vi "Cursors Page.vi"() -> ()   [LabVIEW 2020, in "2D Plot.lvclass"]
uses:
  <vilib>/Math Plots/2D Math Plots/2D Plot/2D Plot/2D Plot.lvclass
  <vilib>/Math Plots/2D Math Plots/2D Plot/Action String/2DMathPlot Ctrl Act Queue.ctl
  <vilib>/Math Plots/2D Math Plots/2D Plot/Action String/2DMathPlot Ctrl Act Cluster.ctl
  <vilib>/Math Plots/2D Math Plots/2D Plot/Action String/2DMathPlot State Class.ctl
  <vilib>/Math Plots/2D Math Plots/2D Plot/2D Plot/Typedef/Cursor Property.ctl
  <vilib>/Utility/miscctls.llb/LVCursorListTypeDef.ctl
  <vilib>/Math Plots/2D Math Plots/2D Plot/2D Plot/Typedef/Dialog State.ctl
  <vilib>/Math Plots/2D Math Plots/2D Plot/2D Plot/Typedef/Temp Graph State.ctl
panel:
  in  "Cursor":string="Cursors"
  in  "Plot # Prefix":string="All Plots"
  out "Cursor Property Out":T1
  in  "Cursor Property In":T1
  in  "Control Ref Queue":T3
  in  "Event Registration":refnum<event-registration>
  in  "Show Cursor":bool caption="Show name"
  in  "Line Width":T4 caption="Cursor Line Width"
  in  "Point Style":T5 caption="Cursor Point Style"
  in  "Line Style":T6 caption="Cursor Line Style"
  in  "Plot #":i32(ring) caption="Plot.Point Style" items=["All Plots", "Plot 0", ""]
  in  "Locking":i32(ring) caption="Plot.Line Width" items=["Free dragging", "Single-plot", "Multi-plot"]
  in  "Delete":bool
  in  "Add":bool
  in  "Show Name":bool caption="Show name"
  in  "Allow Dragging":bool caption="Allow dragging"
  in  "Cursor Name":string caption="Name"
  in  "Cursor Style":T7
  in  "Cursor Color":u32(colorbox) caption="Cursor color"
  in  "Active Cursor":i32(ring) caption="xActive Cursor"
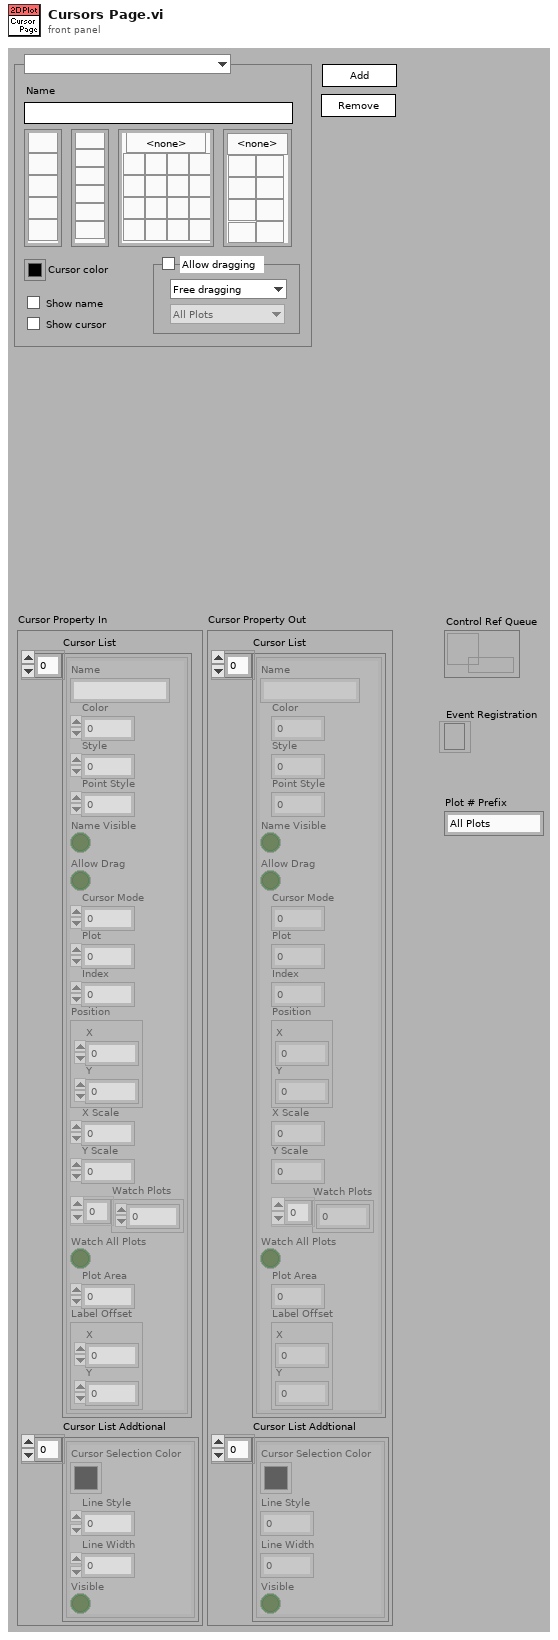
[diagram p1: front panel]
types:
  T1 = typedef "2D Plot.lvclass/Cursor Property.ctl" = cluster{"Cursor List":T2, "Cursor List Addtional":cluster{"Cursor Selection Color":u32, "Line Style":u8, "Line Width":u8, "Visible":bool}[]}
  T2 = typedef "LVCursorListTypeDef.ctl" = cluster{"Name":string, "Color":u32, "Style":u8, "Point Style":u8, "Name Visible":bool, "Allow Drag":bool, "Cursor Mode":u32, "Plot":i32, "Index":i32, "Position":cluster{"X":dbl, "Y":dbl}, "X Scale":u32, "Y Scale":u32, "Watch Plots":i32[], "Watch All Plots":bool, "Plot Area":i32, "Label Offset":cluster{"X":dbl, "Y":dbl}}[]
  T3 = typedef "2DMathPlot Ctrl Act Queue.ctl" = refnum<queue>
  T4 = cluster{"OK Button 2":bool, "OK Button 3":bool, "OK Button 4":bool, "OK Button 5":bool, "OK Button 6":bool, "OK Button 7":bool}
  T5 = cluster{"OK Button 17":bool, "OK Button":bool, "OK Button 2":bool, "OK Button 3":bool, "OK Button 4":bool, "OK Button 5":bool, "OK Button 6":bool, "OK Button 7":bool, "OK Button 8":bool, "OK Button 9":bool, "OK Button 10":bool, "OK Button 11":bool, "OK Button 12":bool, "OK Button 13":bool, "OK Button 14":bool, "OK Button 15":bool, "OK Button 16":bool}
  T6 = cluster{"OK Button":bool, "OK Button 2":bool, "OK Button 3":bool, "OK Button 4":bool, "OK Button 5":bool}
  T7 = cluster{"OK Button 17":bool, "OK Button":bool, "OK Button 2":bool, "OK Button 5":bool, "OK Button 13":bool, "OK Button 10":bool, "OK Button 6":bool, "OK Button 9":bool, "OK Button 14":bool}
  T8 = typedef "2D Plot.lvclass/Dialog State.ctl" = enum16{"Initialize", "Read Property", "Write Property", "Idle", "Exit"}
  T9 = typedef "2DMathPlot Ctrl Act Cluster.ctl" = cluster{"Plot Area Ref":refnum<vi>, "Z Axis Ref":refnum<vi>, "Legend Ref":refnum<vi>, "XControl Ref":refnum<vi>, "Facade Ref":refnum<vi>, "Display State Change Class":T10}
  T10 = typedef "2DMathPlot State Class.ctl" = enum16{"Update All (Undo)", "Update General", "Update Appearance", "Update Format", "Update Scale", "Update Marker", "Update Cursor", "None"}
  T11 = typedef "2D Plot.lvclass/Temp Graph State.ctl" = enum16{"Create", "Update Graph", "Update Property Only", "Get Plot Name", "Get Axis Name", "Destory"}
  T12 = cluster{"Cursor Selection Color":u32, "Line Style":u8, "Line Width":u8, "Visible":bool}
  T13 = cluster{"Name":string, "Color":u32, "Style":u8, "Point Style":u8, "Name Visible":bool, "Allow Drag":bool, "Cursor Mode":u32, "Plot":i32, "Index":i32, "Position":cluster{"X":dbl, "Y":dbl}, "X Scale":u32, "Y Scale":u32, "Watch Plots":i32[], "Watch All Plots":bool, "Plot Area":i32, "Label Offset":cluster{"X":dbl, "Y":dbl}}
  T14 = cluster{"Cursor Selection Color":u32, "Line Style":u8, "Line Width":u8, "Visible":bool}[]
  T15 = cluster{"Bool Array[0]":bool, "Bool Array[1]":bool, "Bool Array[2]":bool, "Bool Array[3]":bool, "Bool Array[4]":bool, "Bool Array[5]":bool, "Bool Array[6]":bool, "Bool Array[7]":bool, "Bool Array[8]":bool, "Bool Array[9]":bool, "Bool Array[10]":bool, "Bool Array[11]":bool, "Bool Array[12]":bool, "Bool Array[13]":bool, "Bool Array[14]":bool, "Bool Array[15]":bool, "Bool Array[16]":bool}
  T16 = cluster{"Bool Array[0]":bool, "Bool Array[1]":bool, "Bool Array[2]":bool, "Bool Array[3]":bool, "Bool Array[4]":bool, "Bool Array[5]":bool, "Bool Array[6]":bool, "Bool Array[7]":bool, "Bool Array[8]":bool}
  T17 = cluster{"Bool Array[0]":bool, "Bool Array[1]":bool, "Bool Array[2]":bool, "Bool Array[3]":bool, "Bool Array[4]":bool}
  T18 = cluster{"Bool Array[0]":bool, "Bool Array[1]":bool, "Bool Array[2]":bool, "Bool Array[3]":bool, "Bool Array[4]":bool, "Bool Array[5]":bool}
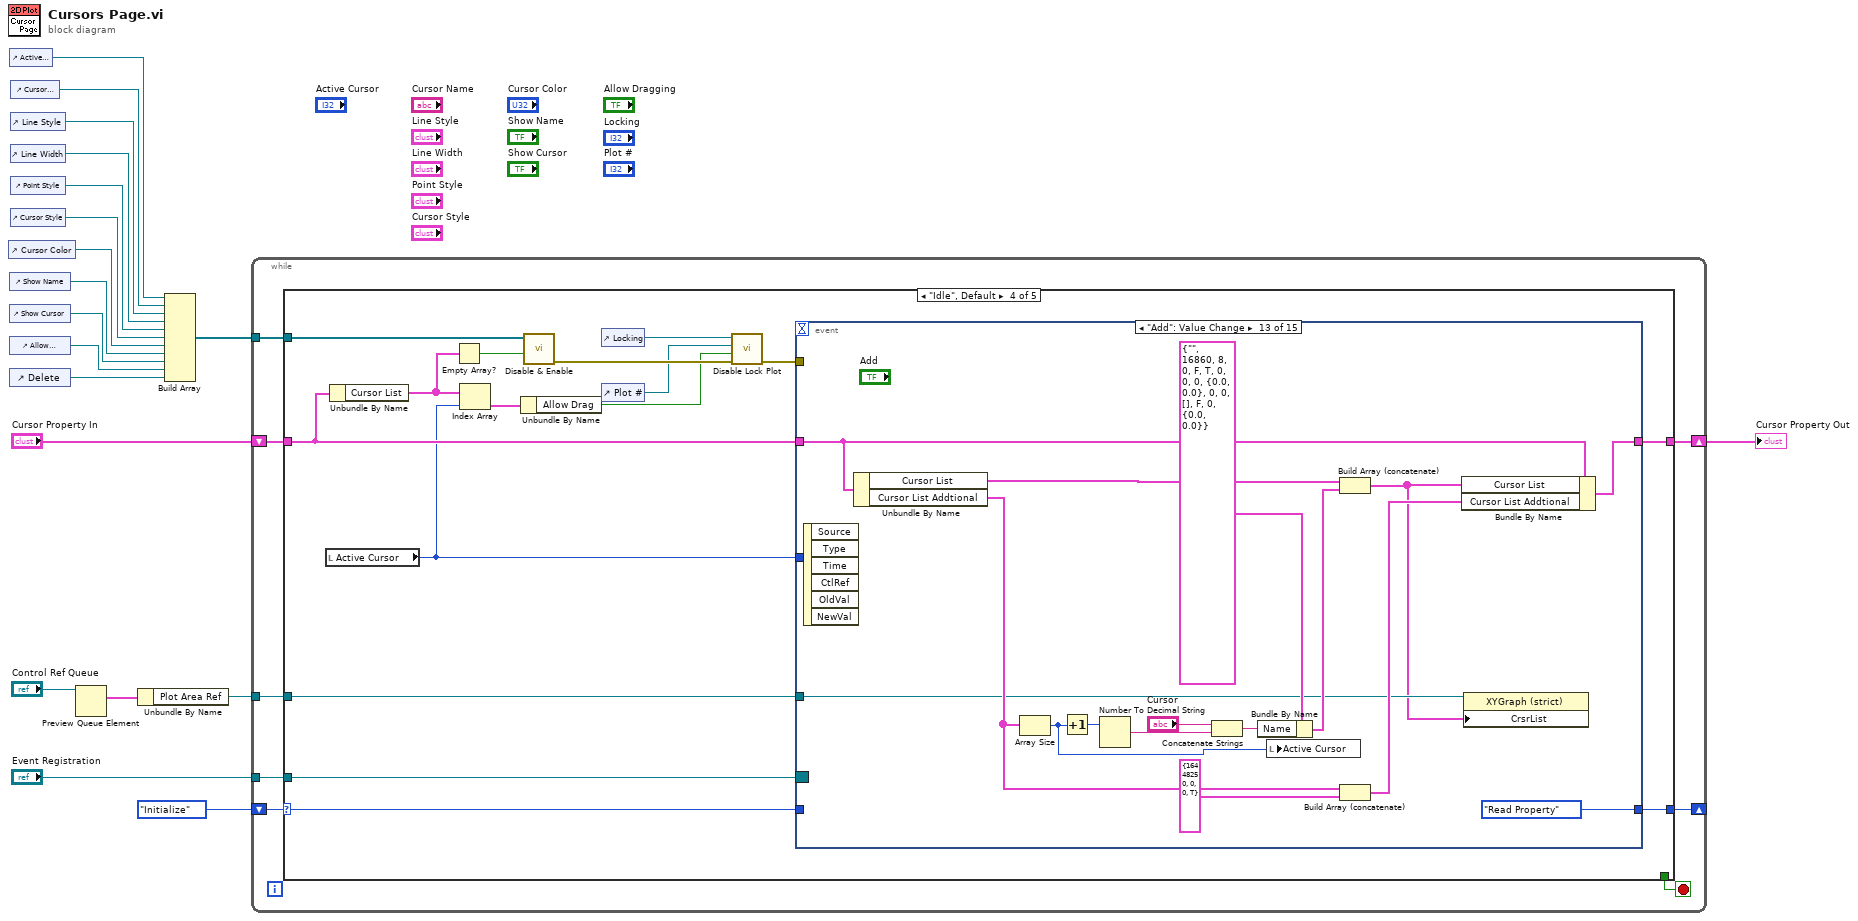
[diagram p0: block diagram]
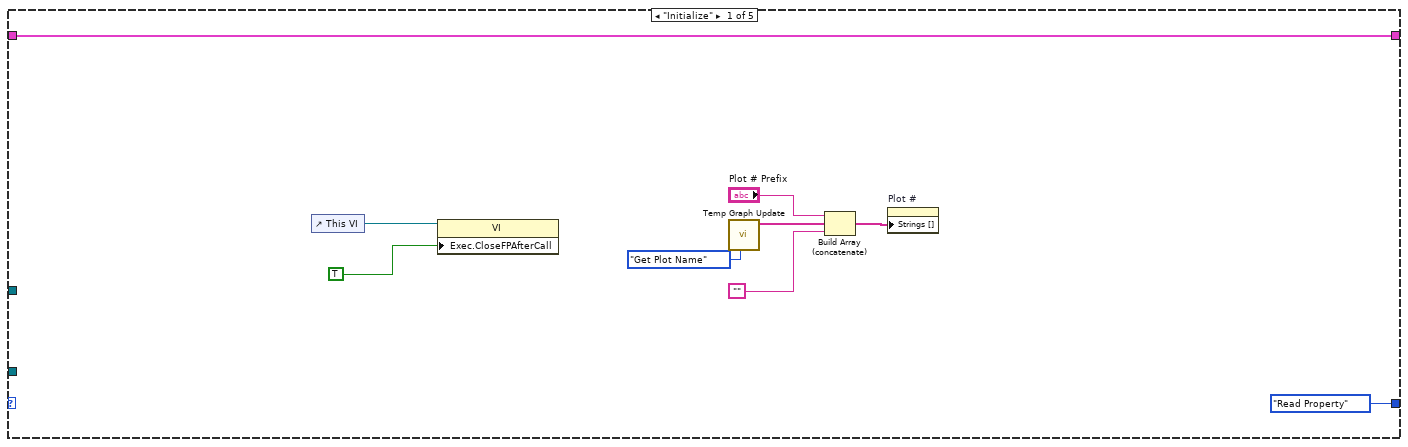
[diagram p2: hidden frame]
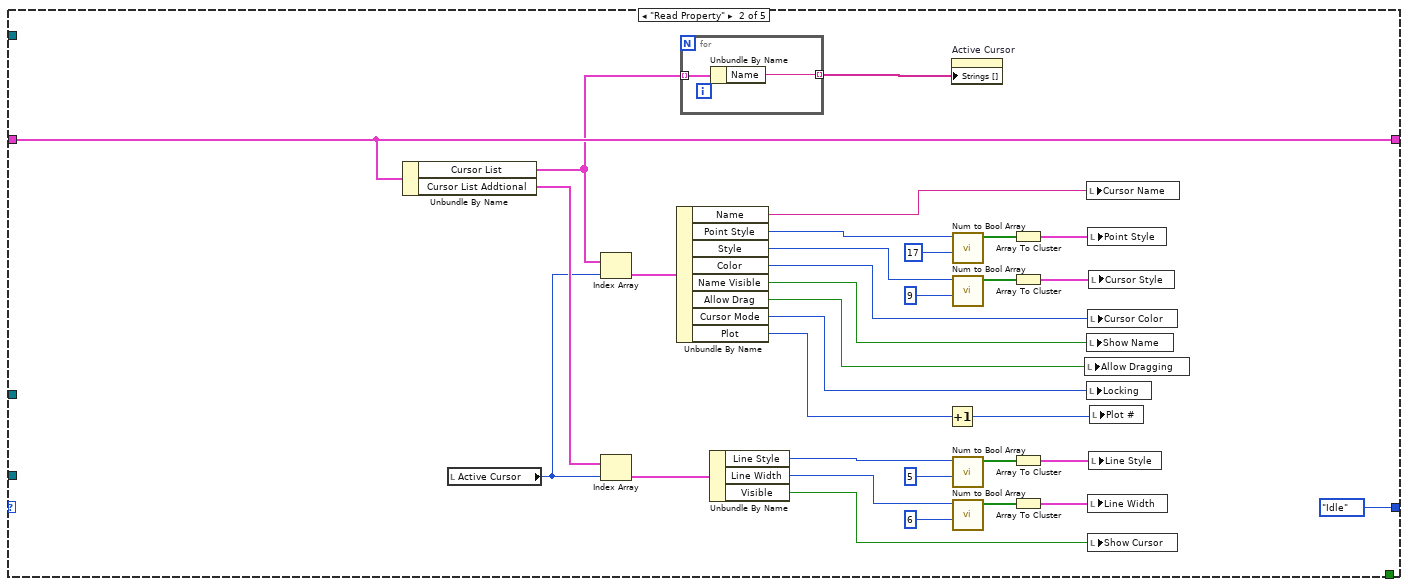
[diagram p3: hidden frame]
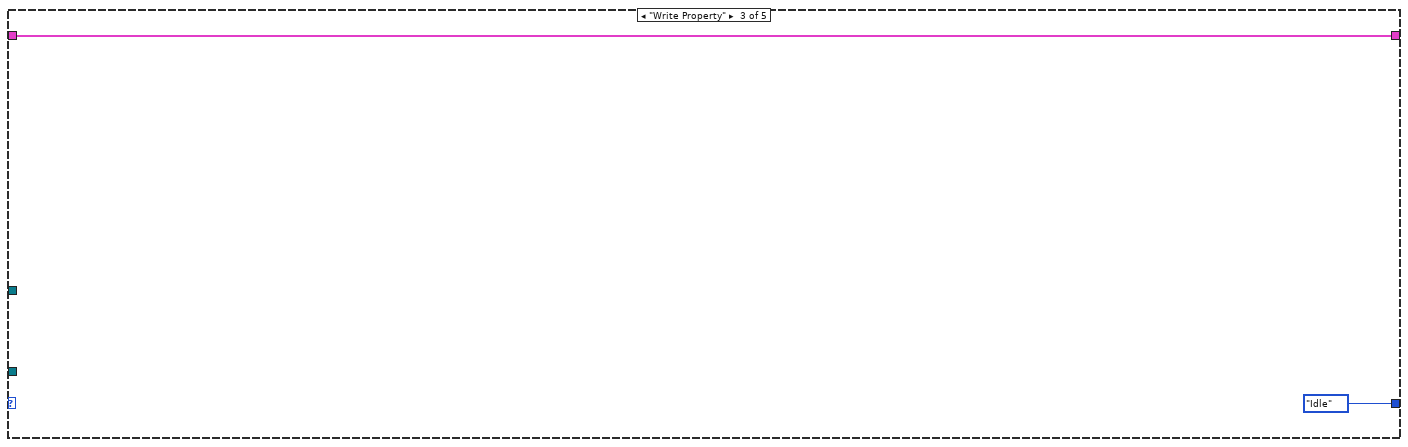
[diagram p4: hidden frame]
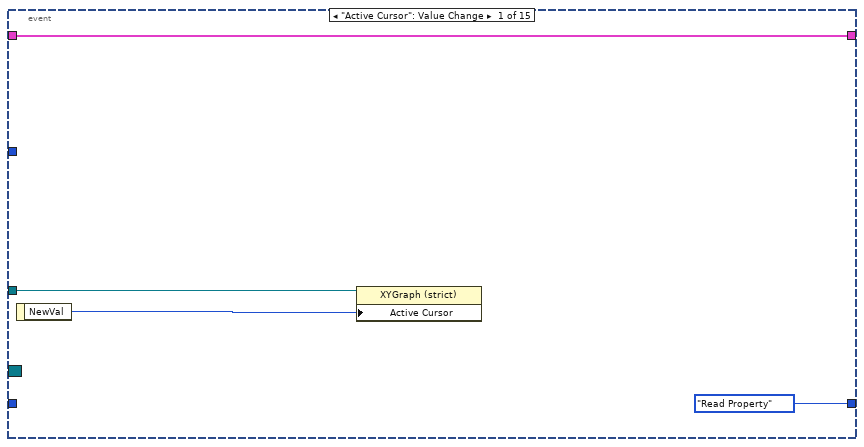
[diagram p5: hidden frame]
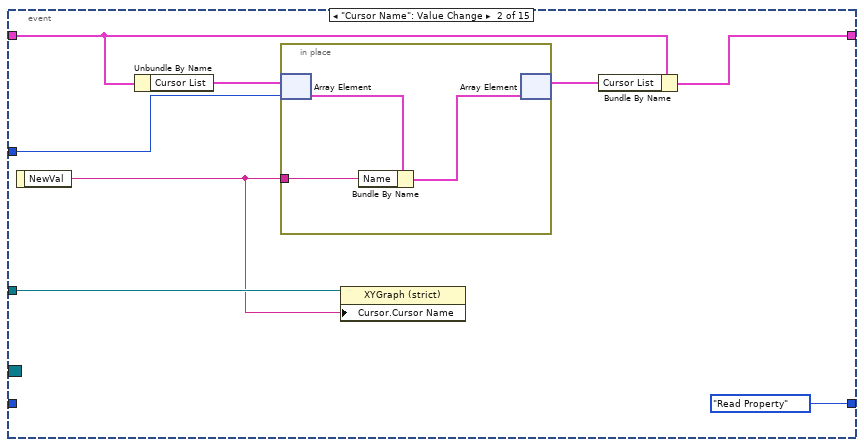
[diagram p6: hidden frame]
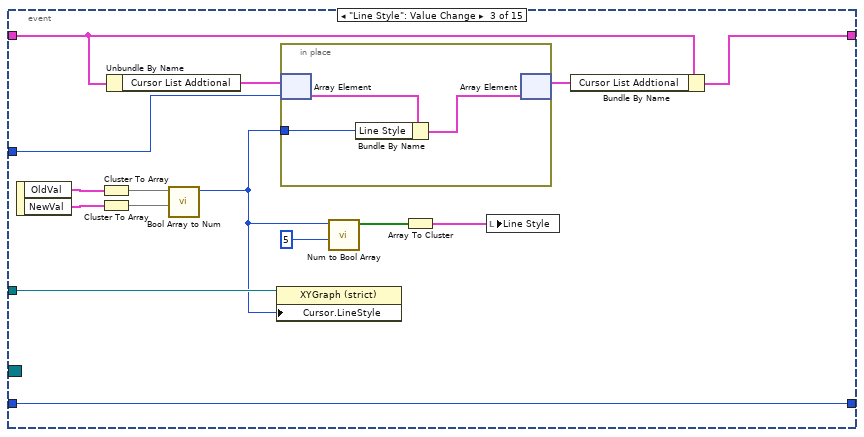
[diagram p7: hidden frame]
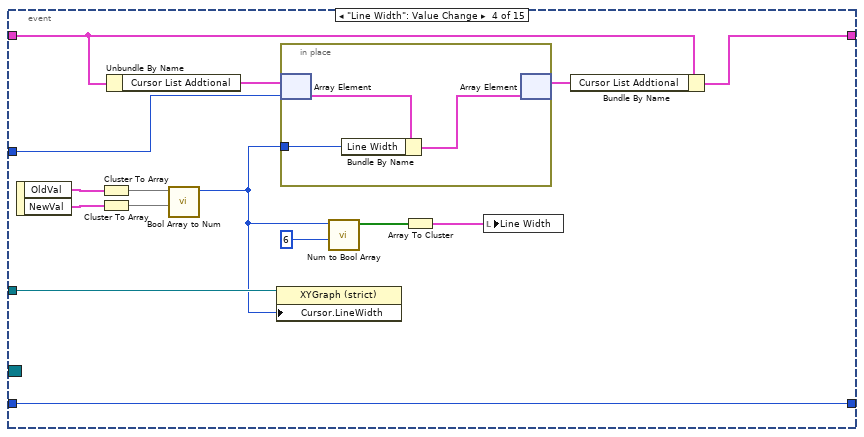
[diagram p8: hidden frame]
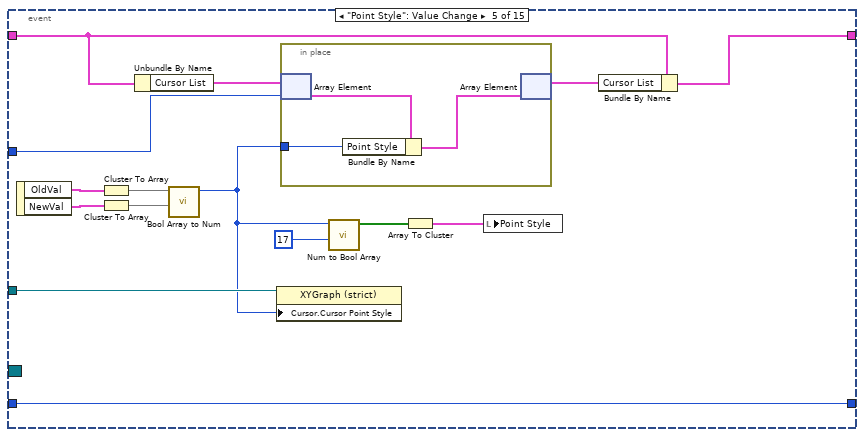
[diagram p9: hidden frame]
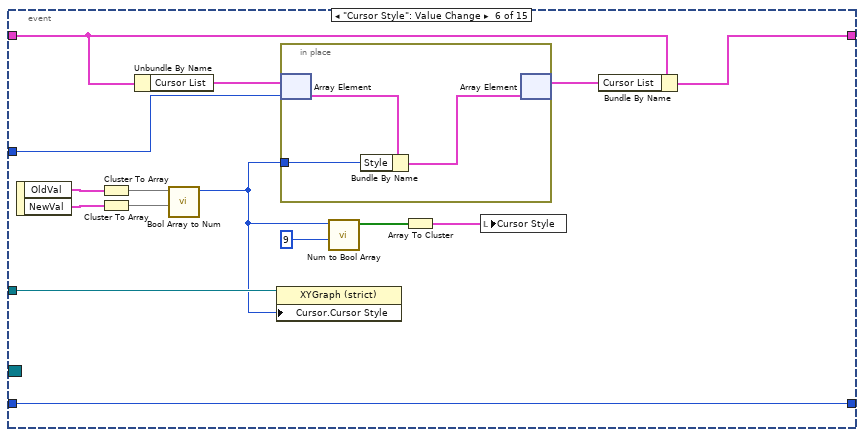
[diagram p10: hidden frame]
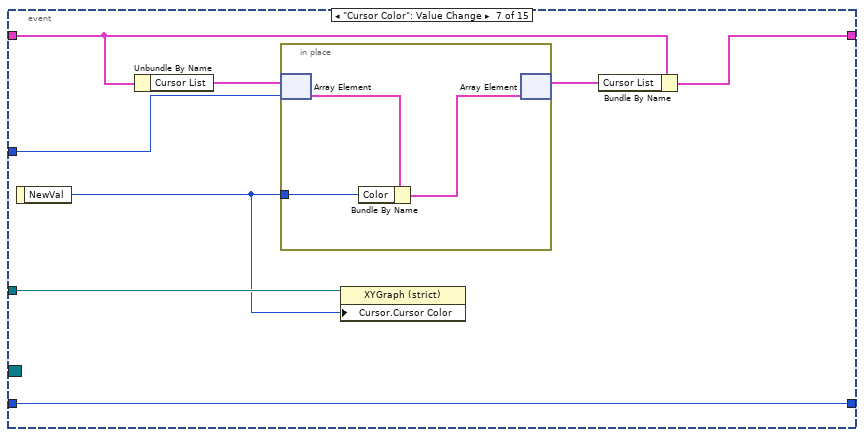
[diagram p11: hidden frame]
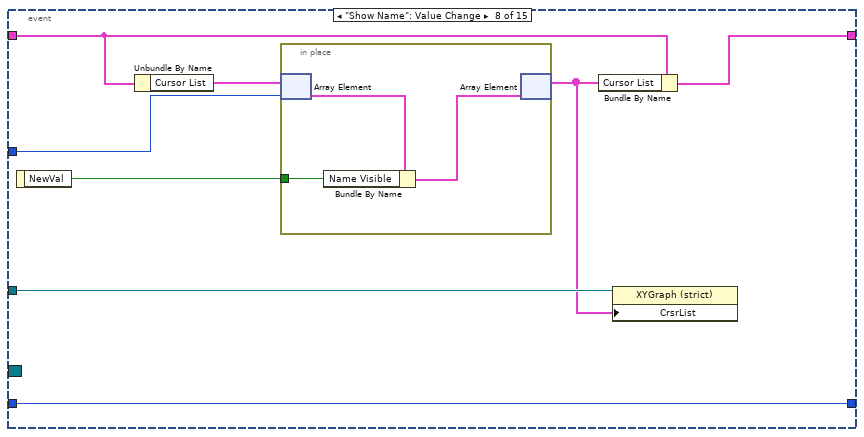
[diagram p12: hidden frame]
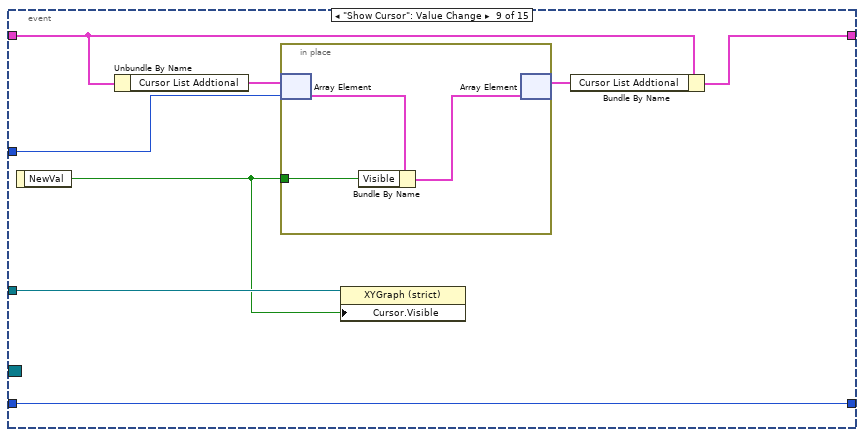
[diagram p13: hidden frame]
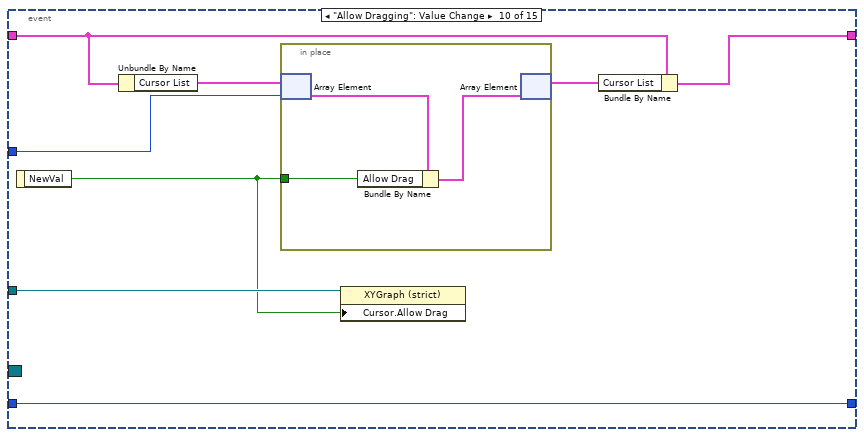
[diagram p14: hidden frame]
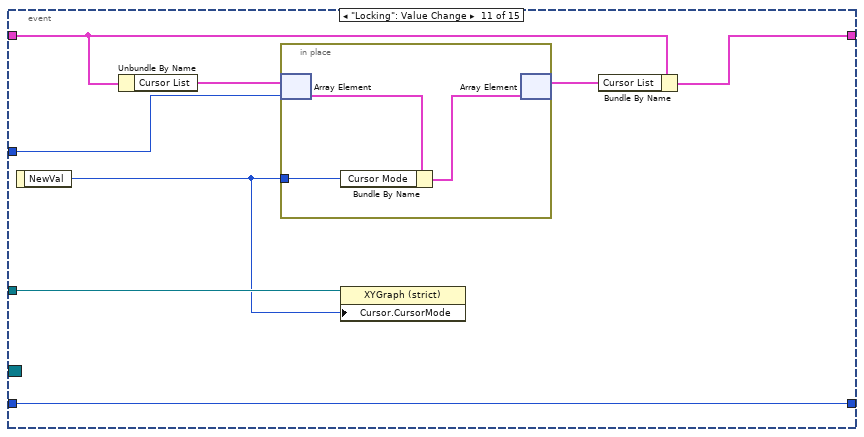
[diagram p15: hidden frame]
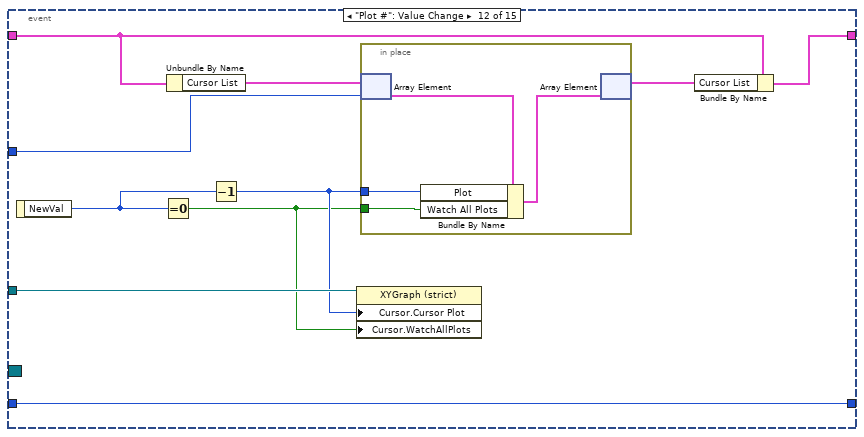
[diagram p16: hidden frame]
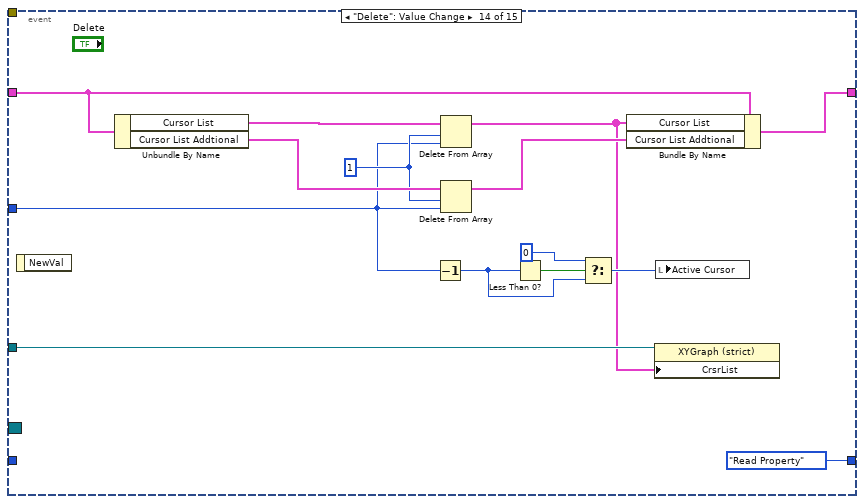
[diagram p17: hidden frame]
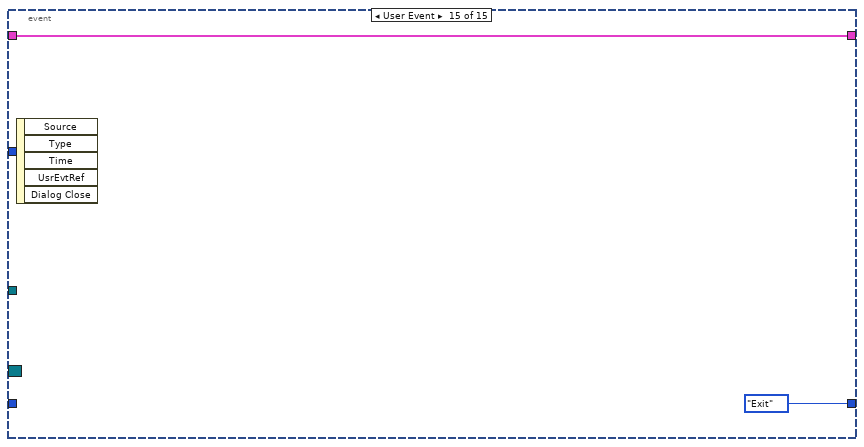
[diagram p18: hidden frame]
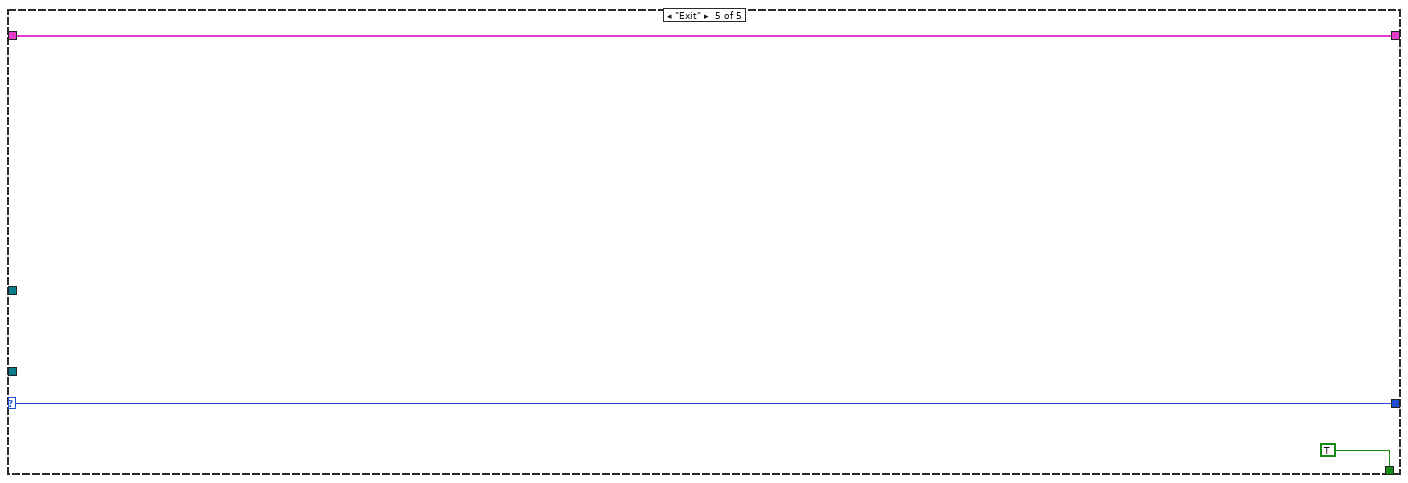
[diagram p19: hidden frame]
diagram:
  n1 = control-ref of="Cursor Color"() -> (w6:refnum<vi>)
  n2 = control-ref of="Active Cursor"() -> (w12:refnum<vi>)
  n3 = control-ref of="Show Name"() -> (w5:refnum<vi>)
  n4 = control-ref of="Show Cursor"() -> (w4:refnum<vi>)
  n5 = control-ref of="Allow Dragging"() -> (w3:refnum<vi>)
  n6 = control-ref of="Delete"() -> (w1:refnum<vi>)
  n7 = control-ref of="Cursor Name"() -> (w11:refnum<vi>)
  n8 = control-ref of="Line Style"() -> (w10:refnum<vi>)
  n9 = control-ref of="Line Width"() -> (w9:refnum<vi>)
  n10 = control-ref of="Point Style"() -> (w8:refnum<vi>)
  n11 = control-ref of="Cursor Style"() -> (w7:refnum<vi>)
  n12 = Preview Queue Element(queue="Control Ref Queue") -> (element=w19:T9)  [unwired: 1 in, 4 out]
  n13 = Unbundle By Name(w19) -> ("Plot Area Ref"=w16:refnum<vi>)
  n14 = Build Array(w12, w11, w10, w9, w8, w7, w6, w5, w4, w3, w1) -> (w2:refnum<vi>[])
  n15 = while {
    shift-right: [w24] -> _
    shift-left: Dialog_State."Initialize" ("Enum") -> [w27]
    tunnel: w16 -> [w26]
    tunnel: "Event Registration" -> [w25]
    shift-right: [w22] -> w13
    shift-left: "Cursor Property In" -> [w23]
    tunnel: w2 -> [w20]
    stop <- w21 stop-if-true
    n16 = case shown="\"Idle\", Default" w27 {
      selector: w27 -> [_ _ _ w84 w278]
      tunnel: w26 -> [_ _ _ w85 _]
      tunnel: w25 -> [_ _ _ w88 _]
      tunnel: [Dialog_State."Read Property" ("Enum") Dialog_State."Idle" ("Enum") Dialog_State."Idle" ("Enum") w87 w278] -> w24
      tunnel: w23 -> [w33 w62 w72 w82 w279]
      tunnel: [w33 w62 w72 w86 w279] -> w22
      tunnel: [_ _ _ _ TRUE] -> w21
      tunnel: w20 -> [_ _ _ w83 _]
      frame "Initialize" {
        n17 = control-ref of="This VI"() -> (w36:refnum<vi>)
        n18 = property class="VI"(reference=w36, "Exec.CloseFPAfterCall"=TRUE ("Execution:Close After Call")) -> ()  [unwired: 1 in, 2 out]
        n19 = call <vilib>:"Temp Graph Update.vi"("State"=Temp_Graph_State."Get Plot Name") -> ("Item Strings"=w29:string[])  [unwired: 4 in, 6 out]
        n20 = Build Array (concatenate)("Plot # Prefix", w29, "") -> (w30:string[])
        n21 = property on="Plot #" class="Ring (strict)"("Strings []"=w30) -> ()  [unwired: 2 in, 2 out]
      }
      frame "Read Property" {
        n22 = Unbundle By Name(w62) -> ("Cursor List"=w61:T2, "Cursor List Addtional"=w60:T14)
        n23 = local read "Active Cursor"() -> (w59:i32)
        n24 = Index Array(array=w61, index=w59) -> (element=w68:T13)
        n25 = Index Array(array=w60, index=w59) -> (element=w58:T12)
        n26 = Unbundle By Name(w68) -> ("Name"=w66:string, "Point Style"=w49:u8, "Style"=w45:u8, "Color"=w44:u32, "Name Visible"=w43:bool, "Allow Drag"=w42:bool, "Cursor Mode"=w41:u32, "Plot"=w39:i32)
        n27 = for {
          tunnel: w61 -> [w70] mode=indexing
          tunnel: [w69] -> w67 mode=indexing
          n28 = Unbundle By Name(w70) -> ("Name"=w69:string)
        }
        n29 = Unbundle By Name(w58) -> ("Line Style"=w57:u8, "Line Width"=w53:u8, "Visible"=w37:bool)
        n30 = Increment(x=w39) -> (x+1=w38:i32)
        n31 = property on="Active Cursor" class="Ring (strict)"("Strings []"=w67) -> ()  [unwired: 2 in, 2 out]
        n32 = call <vilib>:"Num to Bool Array.vi"("Array Size"=17, "Value"=w49) -> ("Bool Array"=w50:bool[])  [unwired: 9 out]
        n33 = call <vilib>:"Num to Bool Array.vi"("Array Size"=9, "Value"=w45) -> ("Bool Array"=w48:bool[])  [unwired: 9 out]
        n34 = call <vilib>:"Num to Bool Array.vi"("Array Size"=5, "Value"=w57) -> ("Bool Array"=w65:bool[])  [unwired: 9 out]
        n35 = call <vilib>:"Num to Bool Array.vi"("Array Size"=6, "Value"=w53) -> ("Bool Array"=w55:bool[])  [unwired: 9 out]
        n36 = Array To Cluster(array=w50) -> (cluster=w51:T15)
        n37 = Array To Cluster(array=w48) -> (cluster=w47:T16)
        n38 = Array To Cluster(array=w65) -> (cluster=w64:T17)
        n39 = Array To Cluster(array=w55) -> (cluster=w54:T18)
        n40 = local write "Allow Dragging"(w42) -> ()
        n41 = local write "Cursor Name"(w66) -> ()
        n42 = local write "Show Name"(w43) -> ()
        n43 = local write "Locking"(w41) -> ()
        n44 = local write "Point Style"(w51) -> ()
        n45 = local write "Cursor Color"(w44) -> ()
        n46 = local write "Line Width"(w54) -> ()
        n47 = local write "Show Cursor"(w37) -> ()
        n48 = local write "Cursor Style"(w47) -> ()
        n49 = local write "Line Style"(w64) -> ()
        n50 = local write "Plot #"(w38) -> ()
      }
      frame "Write Property" {
      }
      frame "Idle", Default {
        n51 = local read "Active Cursor"() -> (w78:i32)
        n52 = Unbundle By Name(w82) -> ("Cursor List"=w80:T2)
        n53 = Empty Array?(array=w80) -> (empty?=w81:bool)
        n54 = Index Array(array=w80, index=w78) -> (element=w79:T13)
        n55 = Unbundle By Name(w79) -> ("Allow Drag"=w76:bool)
        n56 = call <vilib>:"Disable & Enable.vi"("Disabled?"=w81, "Control Ref Array"=w83) -> ("error out"=w77:errorcluster)  [unwired: 1 in, 8 out]
        n57 = control-ref of="Locking"() -> (w75:refnum<vi>)
        n58 = control-ref of="Plot #"() -> (w74:refnum<vi>)
        n59 = call <vilib>:"Disable Lock Plot.vi"("error in (no error)"=w77, "Allow Drag"=w76, "Plot # Refnum"=w74, "Locking Refnum"=w75) -> ("error out"=w73:errorcluster)  [unwired: 7 out]
        n60 = event shown="[12] \"Add\": Value Change" {
          selector: w88 -> [_ _ _ _ _ _ _ _ _ _ _ _ _ _ _]
          dyn-events: _ -> [_ _ _ _ _ _ _ _ _ _ _ _ _ _ _]
          timeout: _ -> [_ _ _ _ _ _ _ _ _ _ _ _ _ _ _]
          tunnel: w82 -> [w91 w99 w117 w135 w153 w171 w182 w193 w204 w215 w226 w239 w259 w274 w276]
          tunnel: [Dialog_State."Read Property" ("Enum") Dialog_State."Read Property" ("Enum") w105 w123 w141 w159 w177 w191 w199 w210 w221 w235 Dialog_State."Read Property" ("Enum") Dialog_State."Read Property" ("Enum") Dialog_State."Exit" ("Enum")] -> w87
          tunnel: [w91 w97 w115 w133 w151 w169 w180 w192 w202 w213 w224 w237 w257 w273 w276] -> w86
          tunnel: w85 -> [w90 w96 w114 w132 w150 w168 w179 w188 w201 w212 w223 w236 w248 w262 _]
          tunnel: w84 -> [_ _ w105 w123 w141 w159 w177 w191 w199 w210 w221 w235 _ _ _]
          tunnel: w78 -> [_ w94 w104 w122 w140 w158 w176 w190 w198 w209 w220 w234 _ w264 _]
          tunnel: w73 -> [_ _ _ _ _ _ _ _ _ _ _ _ _ _ _]
          event "Active Cursor": Value Change {
            n61 = event-data() -> ("NewVal"=w89:i32)  [unwired: 1 out]
            n62 = property class="XYGraph (strict)"(reference=w90, "Active Cursor"=w89) -> ()  [unwired: 1 in, 2 out]
          }
          event "Cursor Name": Value Change {
            n63 = event-data() -> ("NewVal"=w95:string)  [unwired: 1 out]
            n64 = Unbundle By Name(w99) -> ("Cursor List"=w100:T2)
            n65 = in-place {
              in-place-border: w95 -> [w101]
              n66 = in-place-array #1(w100, w94) -> (w103:T13)
              n67 = Bundle By Name(cluster=w103, "Name"=w101) -> (w102:T13)
              n68 = in-place-array #1(w102) -> (w98:T2)  [unwired: 1 out]
            }
            n69 = property class="XYGraph (strict)"(reference=w96, "Cursor.Cursor Name"=w95) -> ()  [unwired: 1 in, 2 out]
            n70 = Bundle By Name(cluster=w99, "Cursor List"=w98) -> (w97:T1)
          }
          event "Line Style": Value Change {
            n71 = event-data() -> ("OldVal"=w113:T6, "NewVal"=w112:T6)  [unwired: 1 out]
            n72 = Cluster To Array(cluster=w113) -> (array=w110:bool[])
            n73 = Cluster To Array(cluster=w112) -> (array=w111:bool[])
            n74 = Unbundle By Name(w117) -> ("Cursor List Addtional"=w118:T14)
            n75 = call <vilib>:"Bool Array to Num.vi"("New Bool Array"=w111, "Old Bool Array"=w110) -> ("Value"=w109:u8)  [unwired: 9 out]
            n76 = property class="XYGraph (strict)"(reference=w114, "Cursor.LineStyle"=w109) -> ()  [unwired: 1 in, 2 out]
            n77 = in-place {
              in-place-border: w109 -> [w119]
              n78 = in-place-array #2(w118, w104) -> (w121:T12)
              n79 = Bundle By Name(cluster=w121, "Line Style"=w119) -> (w120:T12)
              n80 = in-place-array #2(w120) -> (w116:T14)  [unwired: 1 out]
            }
            n81 = call <vilib>:"Num to Bool Array.vi"("Array Size"=5, "Value"=w109) -> ("Bool Array"=w107:bool[])  [unwired: 9 out]
            n82 = Array To Cluster(array=w107) -> (cluster=w106:T17)
            n83 = local write "Line Style"(w106) -> ()
            n84 = Bundle By Name(cluster=w117, "Cursor List Addtional"=w116) -> (w115:T1)
          }
          event "Line Width": Value Change {
            n85 = event-data() -> ("OldVal"=w131:T4, "NewVal"=w130:T4)  [unwired: 1 out]
            n86 = Cluster To Array(cluster=w131) -> (array=w128:bool[])
            n87 = Cluster To Array(cluster=w130) -> (array=w129:bool[])
            n88 = Unbundle By Name(w135) -> ("Cursor List Addtional"=w136:T14)
            n89 = call <vilib>:"Bool Array to Num.vi"("New Bool Array"=w129, "Old Bool Array"=w128) -> ("Value"=w127:u8)  [unwired: 9 out]
            n90 = property class="XYGraph (strict)"(reference=w132, "Cursor.LineWidth"=w127) -> ()  [unwired: 1 in, 2 out]
            n91 = in-place {
              in-place-border: w127 -> [w137]
              n92 = in-place-array #3(w136, w122) -> (w139:T12)
              n93 = Bundle By Name(cluster=w139, "Line Width"=w137) -> (w138:T12)
              n94 = in-place-array #3(w138) -> (w134:T14)  [unwired: 1 out]
            }
            n95 = call <vilib>:"Num to Bool Array.vi"("Array Size"=6, "Value"=w127) -> ("Bool Array"=w125:bool[])  [unwired: 9 out]
            n96 = Array To Cluster(array=w125) -> (cluster=w124:T18)
            n97 = local write "Line Width"(w124) -> ()
            n98 = Bundle By Name(cluster=w135, "Cursor List Addtional"=w134) -> (w133:T1)
          }
          event "Point Style": Value Change {
            n99 = event-data() -> ("OldVal"=w149:T5, "NewVal"=w148:T5)  [unwired: 1 out]
            n100 = Cluster To Array(cluster=w149) -> (array=w146:bool[])
            n101 = Cluster To Array(cluster=w148) -> (array=w147:bool[])
            n102 = Unbundle By Name(w153) -> ("Cursor List"=w154:T2)
            n103 = call <vilib>:"Bool Array to Num.vi"("New Bool Array"=w147, "Old Bool Array"=w146) -> ("Value"=w145:u8)  [unwired: 9 out]
            n104 = property class="XYGraph (strict)"(reference=w150, "Cursor.Cursor Point Style"=w145) -> ()  [unwired: 1 in, 2 out]
            n105 = in-place {
              in-place-border: w145 -> [w155]
              n106 = in-place-array #4(w154, w140) -> (w157:T13)
              n107 = Bundle By Name(cluster=w157, "Point Style"=w155) -> (w156:T13)
              n108 = in-place-array #4(w156) -> (w152:T2)  [unwired: 1 out]
            }
            n109 = call <vilib>:"Num to Bool Array.vi"("Array Size"=17, "Value"=w145) -> ("Bool Array"=w143:bool[])  [unwired: 9 out]
            n110 = Array To Cluster(array=w143) -> (cluster=w142:T15)
            n111 = local write "Point Style"(w142) -> ()
            n112 = Bundle By Name(cluster=w153, "Cursor List"=w152) -> (w151:T1)
          }
          event "Cursor Style": Value Change {
            n113 = event-data() -> ("OldVal"=w167:T7, "NewVal"=w166:T7)  [unwired: 1 out]
            n114 = Cluster To Array(cluster=w167) -> (array=w164:bool[])
            n115 = Cluster To Array(cluster=w166) -> (array=w165:bool[])
            n116 = Unbundle By Name(w171) -> ("Cursor List"=w172:T2)
            n117 = call <vilib>:"Bool Array to Num.vi"("New Bool Array"=w165, "Old Bool Array"=w164) -> ("Value"=w160:u8)  [unwired: 9 out]
            n118 = property class="XYGraph (strict)"(reference=w168, "Cursor.Cursor Style"=w160) -> ()  [unwired: 1 in, 2 out]
            n119 = in-place {
              in-place-border: w160 -> [w173]
              n120 = in-place-array #5(w172, w158) -> (w175:T13)
              n121 = Bundle By Name(cluster=w175, "Style"=w173) -> (w174:T13)
              n122 = in-place-array #5(w174) -> (w170:T2)  [unwired: 1 out]
            }
            n123 = call <vilib>:"Num to Bool Array.vi"("Array Size"=9, "Value"=w160) -> ("Bool Array"=w162:bool[])  [unwired: 9 out]
            n124 = Array To Cluster(array=w162) -> (cluster=w161:T16)
            n125 = local write "Cursor Style"(w161) -> ()
            n126 = Bundle By Name(cluster=w171, "Cursor List"=w170) -> (w169:T1)
          }
          event "Cursor Color": Value Change {
            n127 = event-data() -> ("NewVal"=w178:u32)  [unwired: 1 out]
            n128 = Unbundle By Name(w182) -> ("Cursor List"=w183:T2)
            n129 = in-place {
              in-place-border: w178 -> [w184]
              n130 = in-place-array #6(w183, w176) -> (w186:T13)
              n131 = Bundle By Name(cluster=w186, "Color"=w184) -> (w185:T13)
              n132 = in-place-array #6(w185) -> (w181:T2)  [unwired: 1 out]
            }
            n133 = property class="XYGraph (strict)"(reference=w179, "Cursor.Cursor Color"=w178) -> ()  [unwired: 1 in, 2 out]
            n134 = Bundle By Name(cluster=w182, "Cursor List"=w181) -> (w180:T1)
          }
          event "Show Name": Value Change {
            n135 = event-data() -> ("NewVal"=w189:bool)  [unwired: 1 out]
            n136 = Unbundle By Name(w193) -> ("Cursor List"=w194:T2)
            n137 = in-place {
              in-place-border: w189 -> [w195]
              n138 = in-place-array #7(w194, w190) -> (w197:T13)
              n139 = Bundle By Name(cluster=w197, "Name Visible"=w195) -> (w196:T13)
              n140 = in-place-array #7(w196) -> (w187:T2)  [unwired: 1 out]
            }
            n141 = Bundle By Name(cluster=w193, "Cursor List"=w187) -> (w192:T1)
            n142 = property class="XYGraph (strict)"(reference=w188, "CrsrList"=w187) -> ()  [unwired: 1 in, 2 out]
          }
          event "Show Cursor": Value Change {
            n143 = event-data() -> ("NewVal"=w200:bool)  [unwired: 1 out]
            n144 = Unbundle By Name(w204) -> ("Cursor List Addtional"=w205:T14)
            n145 = in-place {
              in-place-border: w200 -> [w206]
              n146 = in-place-array #8(w205, w198) -> (w208:T12)
              n147 = Bundle By Name(cluster=w208, "Visible"=w206) -> (w207:T12)
              n148 = in-place-array #8(w207) -> (w203:T14)  [unwired: 1 out]
            }
            n149 = property class="XYGraph (strict)"(reference=w201, "Cursor.Visible"=w200) -> ()  [unwired: 1 in, 2 out]
            n150 = Bundle By Name(cluster=w204, "Cursor List Addtional"=w203) -> (w202:T1)
          }
          event "Allow Dragging": Value Change {
            n151 = event-data() -> ("NewVal"=w211:bool)  [unwired: 1 out]
            n152 = Unbundle By Name(w215) -> ("Cursor List"=w216:T2)
            n153 = in-place {
              in-place-border: w211 -> [w217]
              n154 = in-place-array #9(w216, w209) -> (w219:T13)
              n155 = Bundle By Name(cluster=w219, "Allow Drag"=w217) -> (w218:T13)
              n156 = in-place-array #9(w218) -> (w214:T2)  [unwired: 1 out]
            }
            n157 = property class="XYGraph (strict)"(reference=w212, "Cursor.Allow Drag"=w211) -> ()  [unwired: 1 in, 2 out]
            n158 = Bundle By Name(cluster=w215, "Cursor List"=w214) -> (w213:T1)
          }
          event "Locking": Value Change {
            n159 = event-data() -> ("NewVal"=w222:i32)  [unwired: 1 out]
            n160 = Unbundle By Name(w226) -> ("Cursor List"=w227:T2)
            n161 = in-place {
              in-place-border: w222 -> [w228]
              n162 = in-place-array #10(w227, w220) -> (w230:T13)
              n163 = Bundle By Name(cluster=w230, "Cursor Mode"=w228) -> (w229:T13)
              n164 = in-place-array #10(w229) -> (w225:T2)  [unwired: 1 out]
            }
            n165 = property class="XYGraph (strict)"(reference=w223, "Cursor.CursorMode"=w222) -> ()  [unwired: 1 in, 2 out]
            n166 = Bundle By Name(cluster=w226, "Cursor List"=w225) -> (w224:T1)
          }
          event "Plot #": Value Change {
            n167 = event-data() -> ("NewVal"=w233:i32)  [unwired: 1 out]
            n168 = Equal To 0?(x=w233) -> (x = 0?=w231:bool)
            n169 = Unbundle By Name(w239) -> ("Cursor List"=w240:T2)
            n170 = Decrement(x=w233) -> (x-1=w232:i32)
            n171 = property class="XYGraph (strict)"(reference=w236, "Cursor.Cursor Plot"=w232, "Cursor.WatchAllPlots"=w231) -> ()  [unwired: 1 in, 2 out]
            n172 = in-place {
              in-place-border: w231 -> [w242]
              in-place-border: w232 -> [w241]
              n173 = in-place-array #11(w240, w234) -> (w244:T13)
              n174 = Bundle By Name(cluster=w244, "Plot"=w241, "Watch All Plots"=w242) -> (w243:T13)
              n175 = in-place-array #11(w243) -> (w238:T2)  [unwired: 1 out]
            }
            n176 = Bundle By Name(cluster=w239, "Cursor List"=w238) -> (w237:T1)
          }
          event "Add": Value Change {
            n177 = event-data() -> ()  [unwired: 7 out]
            n178 = Unbundle By Name(w259) -> ("Cursor List"=w260:T2, "Cursor List Addtional"=w250:T14)
            n179 = Array Size(array=w250) -> (size(s)=w245:i32)
            n180 = Increment(x=w245) -> (x+1=w246:i32)
            n181 = Number To Decimal String(number=w246) -> (decimal integer string=w249:string)  [unwired: 1 out]
            n182 = Concatenate Strings("Cursor", w249) -> (w253:string)
            n183 = Bundle By Name(cluster=T13 {"Name"="", "Color"=16860, "Style"=8, "Point Style"=0, "Name Visible"=FALSE, "Allow Drag"=TRUE, "Cursor Mode"=0, "Plot"=0, "Index"=0, "Position"={"X"=0.0, "Y"=0.0}, "X Scale"=0, "Y Scale"=0, "Watch Plots"=[], "Watch All Plots"=FALSE, "Plot Area"=0, "Label Offset"={"X"=0.0, "Y"=0.0}}, "Name"=w253) -> (w254:T13)
            n184 = local write "Active Cursor"(w245) -> ()
            n185 = Build Array (concatenate)(w260, w254) -> (w247:T2)
            n186 = Build Array (concatenate)(w250, T12 {"Cursor Selection Color"=16448250, "Line Style"=0, "Line Width"=0, "Visible"=TRUE} ("Rest Attribute")) -> (w258:T14)
            n187 = Bundle By Name(cluster=w259, "Cursor List"=w247, "Cursor List Addtional"=w258) -> (w257:T1)
            n188 = property class="XYGraph (strict)"(reference=w248, "CrsrList"=w247) -> ()  [unwired: 1 in, 2 out]
          }
          event "Delete": Value Change {
            w269 = 1 ("length")
            n189 = event-data() -> ()  [unwired: 2 out]
            n190 = Unbundle By Name(w274) -> ("Cursor List"=w272:T2, "Cursor List Addtional"=w271:T14)
            n191 = Decrement(x=w264) -> (x-1=w266:i32)
            n192 = Delete From Array(array=w272, length=w269, index=w264) -> (array with subset deleted=w261:T2)  [unwired: 1 out]
            n193 = Delete From Array(array=w271, length=w269, index=w264) -> (array with subset deleted=w270:T14)  [unwired: 1 out]
            n194 = Less Than 0?(x=w266) -> (x < 0?=w268:bool)
            n195 = Select(t=0, s=w268, f=w266) -> (s? t:f=w265:i32)
            n196 = Bundle By Name(cluster=w274, "Cursor List"=w261, "Cursor List Addtional"=w270) -> (w273:T1)
            n197 = property class="XYGraph (strict)"(reference=w262, "CrsrList"=w261) -> ()  [unwired: 1 in, 2 out]
            n198 = local write "Active Cursor"(w265) -> ()
          }
          event User Event {
            n199 = event-data() -> ()  [unwired: 6 out]
          }
        }
      }
      frame "Exit" {
      }
    }
  }
  "Cursor Property Out" <- w13
